vi "Write Num Of Sliders.vi"(5 "Num Of Sliders":i32, 9 "NumericWithScale in":refnum<class "NumericWithScale.lvclass">) -> (3 "NumericWithScale out":refnum<class "NumericWithScale.lvclass">)   [LabVIEW 2014, in "NumericWithScale.lvclass"]
uses:
  NumericWithScale.lvclass
  NumericWithScale.lvclass/NumericWithScale.ctl
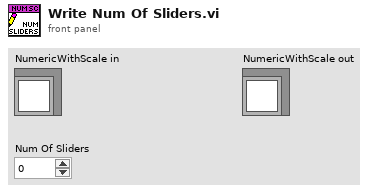
[diagram p1: front panel]
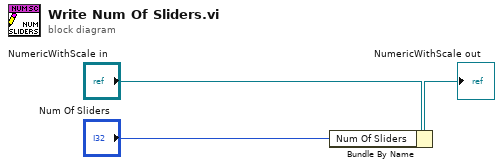
[diagram p0: block diagram]
diagram:
  n1 = Bundle By Name(cluster="NumericWithScale in", "Num Of Sliders"="Num Of Sliders") -> (→"NumericWithScale out":refnum<class "NumericWithScale.lvclass">)
